vi "COM_W_R_No-Termination.vi"(0 "VISA resource name":refnum<visa-resource-name>="COM74", 1 "baud rate":u32=115200, 2 "data bits":u16=8 min=5 max=8 step=1, 3 "parity":u16(ring) items=["None", "Odd", "Even", "Mark", "Space"], 4 "stop bits":u16(ring)=10 items=["1.0"=10, "1.5"=15, "2.0"=20], 5 "write":bool=TRUE, 6 "read":bool=TRUE, 7 "flow control":u16(ring) items=["None"=0, "XON/XOFF"=1, "RTS/CTS"=2, "DTR/DSR"=4], 8 "string to write":string="*IDN?") -> (9 "read string":string)   [LabVIEW 2012]
doc: "The Basic Serial Read and Write example performs a Serial Port Read, a Serial Port Write, or a combination of these actions. The user selects the actions (read or write) on the front panel. If both are selected, the VI will write the data first, read data, and then close the VISA session that is opened to the port. This VI will wait until the specified number of bytes is received at the port. Only the number of bytes specified will be read.\n\nINSTRUCTIONS:\n1) Select the serial resource and configuration parameters (baud rate, data bits, parity, stop bits, flow control).\n2) Select the operations to be performed. \n3) Connect the serial port to your device. If no device is available, perform a loopback test by doing one of the following. Short pins 2 and 3 on a RS-232 cable or short pin 4 to pin 8 and pin 5 to pin 9 on a RS-485/422 cable. \n4) Run the VI to see the data read. (The \"read string\" will match the \"string to write\" if a loopback test was performed.)\n\nNote: The parameters set for the serial port must match the parameters of the connected instrument or device. In this example, the bytes to read parameter specifies the number of bytes that the serial port reads. If there were more bytes at the port than the number specified in bytes to read, those bytes would not be read. Also, if you specify to read more bytes than the number of bytes actually read, you might receive a timeout error message.\n\nOn the block diagram, the Configure Serial Port VI sets the configuration parameters. The front panel displays the controls used to configure the basic parameters, such as baud rate, data bits, and parity. Constants configure the other parameters the user probably does not need set. After the VISA Configure Serial Port VI opens the VISA session and configures the port, the VI passes the VISA resource name to other VIs that perform operations on that VISA resource. The VISA Write function sends a command to the serial device and the VISA Read function returns data based on the command. The VISA Close function then closes the reference to the serial device. It is important to close the reference; otherwise communication through with that port through protocols other than VISA might not be possible."
uses:
  <vilib>/Instr/_visa.llb/VISA Configure Serial Port (Instr).vi
panel:
  out "Bytes at Port":u32
  # "Select the serial resource and the operations (Read, Write, or both) to be performed.  If both are selected, the VI will write the data first, read data and then close the VISA session that is opened to the port.  This VI will wait until the specified number of bytes is received at the port. Only the number of bytes specified will be read."
  # "For additional information select File >> VI Properties >> Documentation"
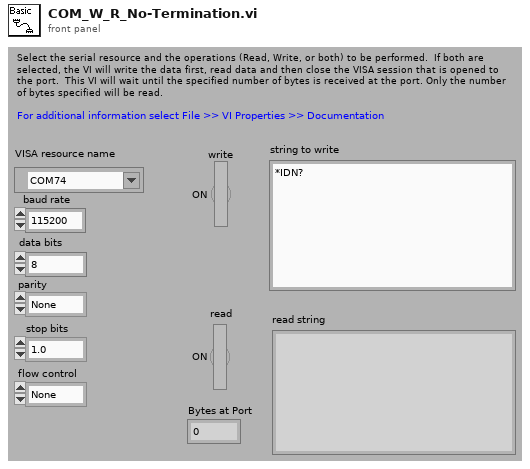
[diagram p1: front panel]
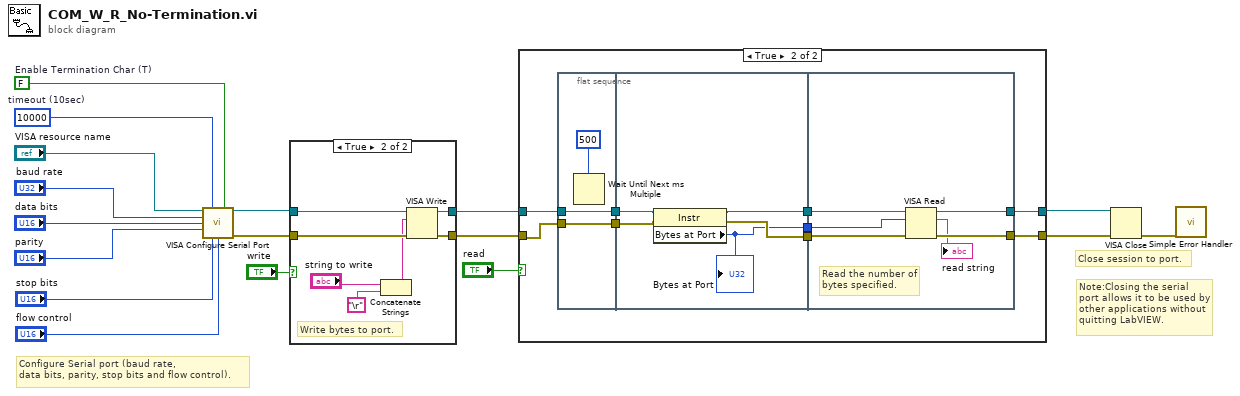
[diagram p0: block diagram]
diagram:
  w9 = FALSE  # Enable Termination Char (T)
  w10 = u32 10000  # timeout (10sec)
  # "Note:Closing the serial port allows it to be used by other applications without\nquitting LabVIEW."
  # "Configure Serial port (baud rate,\ndata bits, parity, stop bits and flow control)."
  # "Close session to port."
  n1 = call-poly "VISA Configure Serial Port"("VISA resource name"="VISA resource name", "timeout (10sec)"=w10, "Enable Termination\nChar (T)"=w9, "baud rate (9600)"="baud rate", "data bits (8)"="data bits", "parity (0:none)"="parity", "stop bits (10: 1 bit)"="stop bits", "flow control (0:none)"="flow control") -> ("VISA resource name out"=w2:refnum<visa-resource-name>, "error out"=w1:errorcluster)  [unwired: 6 in]
  n2 = case shown="True" "write" {
    tunnel: [w19 w26] -> w15
    tunnel: w2 -> [w18 w25]
    tunnel: w1 -> [w19 w24]
    tunnel: [w18 w23] -> w5
    frame False {
    }
    frame True {
      # "Write bytes to port."
      n3 = Concatenate Strings("string to write", "\r") -> (w20:string)
      n4 = VISA Write(VISA resource name=w25, write buffer=w20, error in (no error)=w24) -> (VISA resource name out=w23:refnum<visa-resource-name>, error out=w26:errorcluster)  [unwired: 1 out]
    }
  }
  n5 = case shown="True" "read" {
    tunnel: w15 -> [w28 w34]
    tunnel: [w28 w37] -> w14
    tunnel: [w27 w36] -> w13
    tunnel: w5 -> [w27 w35]
    frame False {
    }
    frame True {
      n6 = flat-sequence {
        tunnel: w34 -> [w38]
        tunnel: w35 -> [w40]
        tunnel: [w40] -> w32
        tunnel: [w38] -> w31
        tunnel: [w42] -> w33
        tunnel: w32 -> [w45]
        tunnel: w31 -> [w44]
        tunnel: [w43] -> w30
        tunnel: [w41] -> w29
        tunnel: [w51] -> w37
        tunnel: [w50] -> w36
        tunnel: w33 -> [w48]
        tunnel: w30 -> [w47]
        tunnel: w29 -> [w46]
        frame #0 {
          n7 = Wait Until Next ms Multiple(millisecond multiple=u32 500) -> ()  [unwired: 1 out]
        }
        frame #1 {
          n8 = property class="Instr"(reference=w45, error in=w44) -> (reference out=w42:refnum<visa-resource-name>, error out=w43:errorcluster, "Bytes at Port"=w41:u32)
          "Bytes at Port" <- w41
        }
        frame #2 {
          # "Read the number of bytes specified."
          n9 = VISA Read(VISA resource name=w48, byte count=w46, error in (no error)=w47) -> (VISA resource name out=w50:refnum<visa-resource-name>, read buffer=→"read string":string, error out=w51:errorcluster)  [unwired: 1 out]
        }
      }
    }
  }
  n10 = VISA Close(VISA resource name=w13, error in (no error)=w14) -> (error out=w12:errorcluster)
  n11 = call <vilib>:"Simple Error Handler.vi"("error in (no error)"=w12) -> ()  [unwired: 4 in, 5 out]
